vi "demo.vi"() -> ()   [LabVIEW 2016]
uses:
  main/apis/Setup/GetVI/GetVIByPath.vi
  main/apis/Stimulus/ValueSignalByPathString.vi
  <vilib>/addons/_JKI Toolkits/Caraya/classes/Test/Test.lvclass
panel:
  out "error out":errorcluster
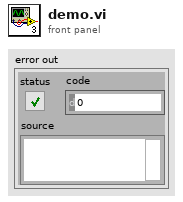
[diagram p1: front panel]
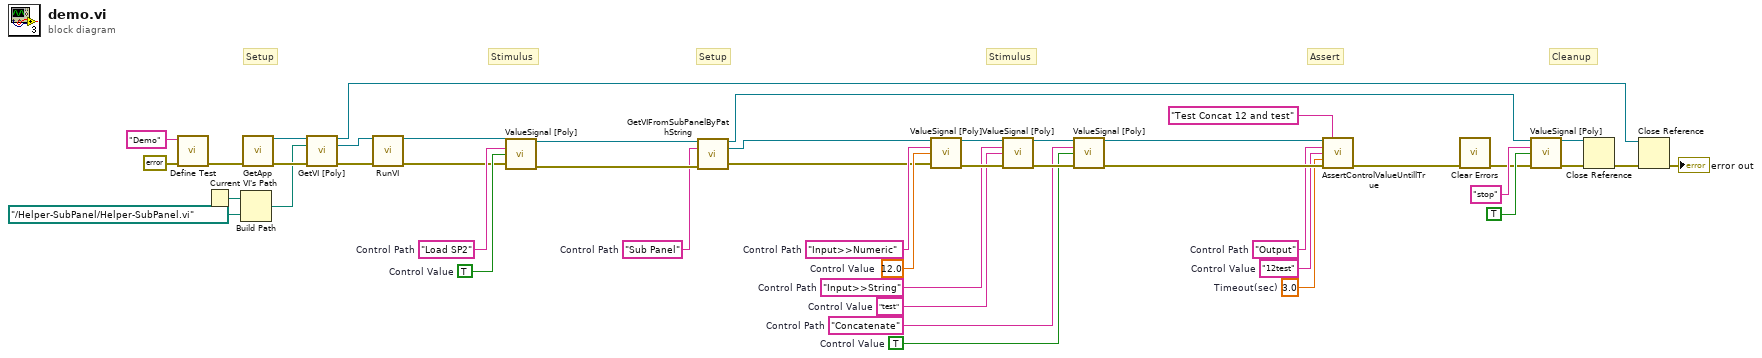
[diagram p0: block diagram]
diagram:
  w14 = "Input>>String"  # Control Path
  w15 = "Sub Panel"  # Control Path
  w20 = 3.0  # Timeout(sec)
  w22 = "12test"  # Control Value
  w23 = "Output"  # Control Path
  w26 = "Input>>Numeric"  # Control Path
  w27 = TRUE  # Control Value
  w28 = "Concatenate"  # Control Path
  w31 = "test"  # Control Value
  w34 = 12.0  # Control Value
  w35 = TRUE  # Control Value
  w36 = "Load SP2"  # Control Path
  # "Cleanup"
  # "Assert"
  # "Setup"
  # "Stimulus"
  # "Stimulus"
  # "Setup"
  n1 = call <vilib>:"Define Test.vi"("error in (no error)"=errorcluster {"status"=FALSE, "code"=0, "source"=""}, "Label (VI Title)"="Demo") -> ("error out"=w44:errorcluster)  [unwired: 9 in]
  n2 = Current VI's Path() -> (path=w9:path)
  n3 = Build Path(base path=w9, name or relative path=path "../Helper-SubPanel/Helper-SubPanel.vi" ("path")) -> (appended path=w10:path)
  n4 = call "GetApp.vi"("error in (no error)"=w44) -> ("Application Ref"=w42:refnum<vi>, "error out"=w41:errorcluster)  [unwired: 13 in]
  n5 = call-poly "GetVI [Poly].vi"("Application Ref in"=w42, "VI Path"=w10, "error in (no error)"=w41) -> ("Application Ref out"=w40:refnum<vi>, "VI Reference"=w5:refnum<vi>, "error out"=w7:errorcluster)  [unwired: 10 in]
  n6 = call "RunVI.vi"("VI Reference In"=w5, "error in"=w7) -> ("VI Reference Out"=w4:refnum<vi>, "error out"=w6:errorcluster)  [unwired: 12 in]
  n7 = call-poly "ValueSignal [Poly].vi"("VI Reference In"=w4, "Control Name"=w36, "Value (Signaling)"=w35, "error in"=w6) -> ("VI Reference Out"=w18:refnum<vi>, "error out"=w19:errorcluster)  [unwired: 10 in]
  n8 = call "GetVIFromSubPanelByPathString.vi"("VI Reference In"=w18, "SubPanel Path"=w15, "error in"=w19) -> ("VI Reference Out"=w13:refnum<vi>, "SubPanel VI Reference"=w16:refnum<vi>, "error out"=w17:errorcluster)  [unwired: 10 in]
  n9 = call-poly "ValueSignal [Poly].vi"("VI Reference In"=w16, "Control Name"=w26, "Value (Signaling)"=w34, "error in"=w17) -> ("VI Reference Out"=w32:refnum<vi>, "error out"=w33:errorcluster)  [unwired: 10 in]
  n10 = call-poly "ValueSignal [Poly].vi"("VI Reference In"=w32, "Control Name"=w14, "Value (Signaling)"=w31, "error in"=w33) -> ("VI Reference Out"=w29:refnum<vi>, "error out"=w30:errorcluster)  [unwired: 10 in]
  n11 = call-poly "ValueSignal [Poly].vi"("VI Reference In"=w29, "Control Name"=w28, "Value (Signaling)"=w27, "error in"=w30) -> ("VI Reference Out"=w24:refnum<vi>, "error out"=w25:errorcluster)  [unwired: 10 in]
  n12 = call "AssertControlValueUntillTrue.vi"("VI Reference In"=w24, "Label"="Test Concat 12 and test", "Control Name"=w23, "Control Value"=w22, "Timeout(5 sec)"=w20, "error out"=w25) -> ("error out 2"=w12:errorcluster)  [unwired: 8 in, 1 out]
  n13 = call <vilib>:"Clear Errors.vi"("error in (no error)"=w12) -> ("error out"=w1:errorcluster)  [unwired: 5 in, 1 out]
  n14 = call-poly "ValueSignal [Poly].vi"("VI Reference In"=w13, "Control Name"="stop" ("Class Name"), "Value (Signaling)"=TRUE, "error in"=w1) -> ("VI Reference Out"=w37:refnum<vi>, "error out"=w38:errorcluster)  [unwired: 10 in]
  n15 = Close Reference(reference=w37, error in (no error)=w38) -> (error out=w39:errorcluster)
  n16 = Close Reference(reference=w40, error in (no error)=w39) -> (error out=→"error out":errorcluster)
